vi "Read Desired Temperature.vi"(11 "Cooler Controller in":refnum<class "Cooler Controller.lvclass">) -> (2 "Desired Temperature":dbl=75.0)   [LabVIEW 2025, in "Cooler Controller.lvlib" / "Cooler Controller.lvclass"]
uses:
  Cooler Controller.lvclass
  Cooler Controller.lvclass/Cooler Controller.ctl
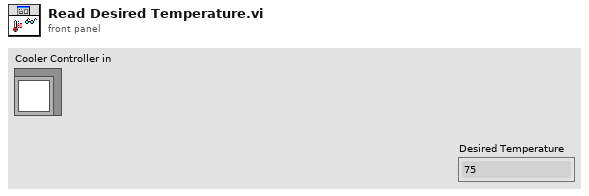
[diagram p1: front panel]
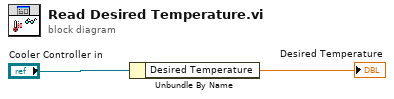
[diagram p0: block diagram]
diagram:
  n1 = Unbundle By Name("Cooler Controller in") -> ("Desired Temperature"=→"Desired Temperature":dbl)
